vi "create.messages.for.testing.vi"(10 "Message.to.Create":refnum<class "MessageBase.lvclass">[](array[class]), 11 "Messages to Create":T1[](array[typedef])) -> (3 "Words.Out":u16[](array[numeric]) format="%.0x")   [LabVIEW 2020]
uses:
  Message.Spec.ctl
  pitch/oldMessageType.ctl
  pitch/AddOrder/AddOrderLong.Parameters.ctl
  pitch/Time/Time.Parameters.ctl
  pitch/SequencedUnitHeader/SequencedUnitHeader.Parameters.ctl
  pitch/ModifyOrder/ModifyOrderLong.Parameters.ctl
  pitch/MessageBase/MessageBase.lvclass
  pitch/SequencedUnitHeader/SequencedUnitHeader.lvclass
  pitch/Time/Time.lvclass
  pitch/AddOrder/AddOrderLong.lvclass
  pitch/ModifyOrder/ModifyOrderLong.lvclass
panel:
  out "size(s)":i32
  out "Remaining Bytes":u8[](array[numeric])
  out "Raw.Bytes.Out":u8[](array[numeric]) format="%.0x"
  out "Bytes.out (Visual)":u8[][](array[numeric]) format="%.0x"
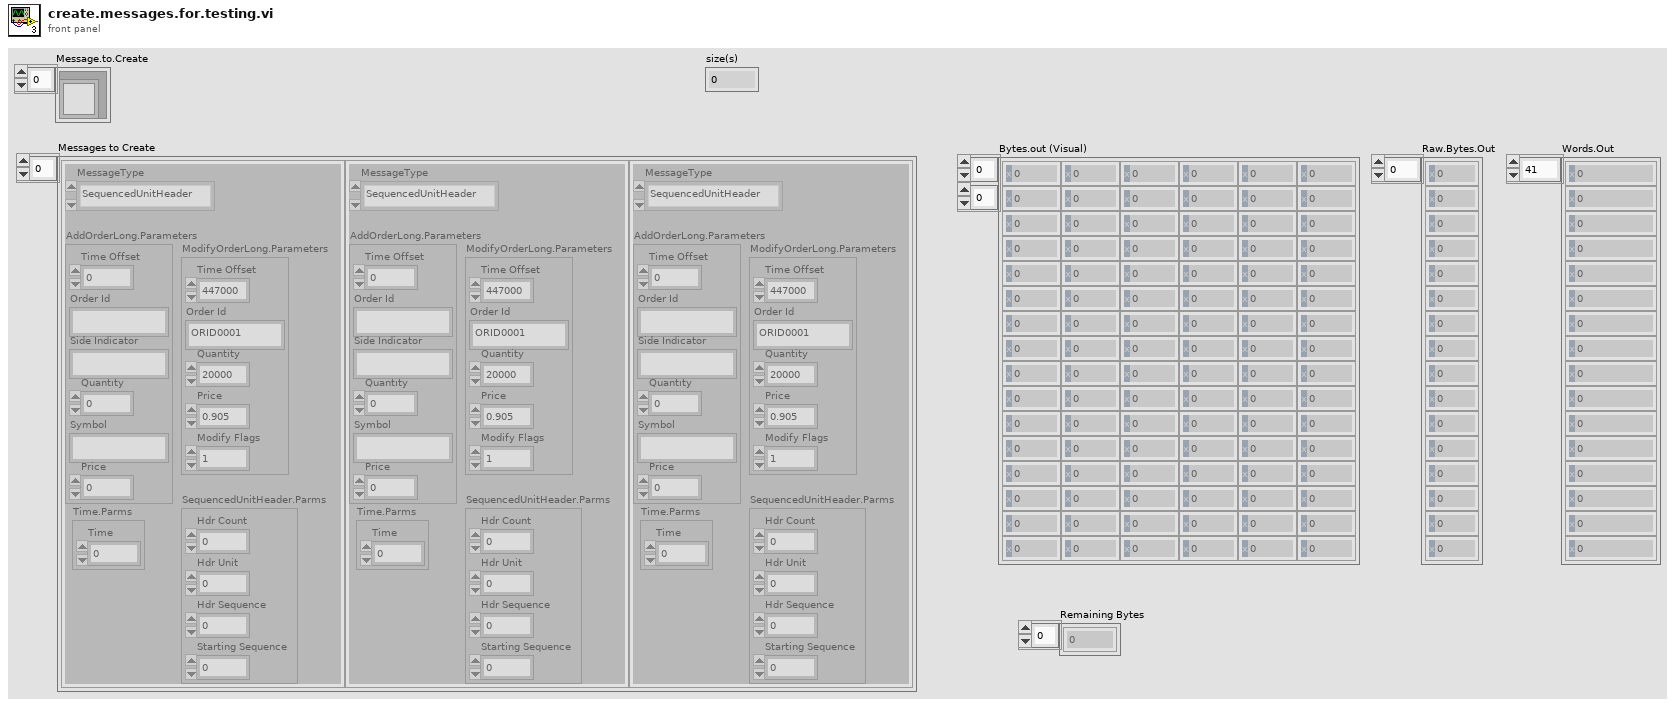
[diagram p1: front panel]
types:
  T1 = typedef "Message.Spec.ctl" = cluster{"MessageType":T2, "AddOrderLong.Parameters":T3, "Time.Parms":T4, "SequencedUnitHeader.Parms":T5, "ModifyOrderLong.Parameters":T6}
  T2 = typedef "oldMessageType.ctl" = enum16{"Time", "SequencedUnitHeader", "AddOrderLong", "AddOrderShort", "AddOrderExpanded", "ModifyOrderLong"}
  T3 = typedef "AddOrderLong.lvclass/AddOrderLong.Parameters.ctl" = cluster{"Time Offset":u32, "Order Id":string, "Quantity":u32, "Symbol":string, "Side Indicator":string, "Price":dbl}
  T4 = typedef "Time.lvclass/Time.Parameters.ctl" = cluster{"Time":u32}
  T5 = typedef "SequencedUnitHeader.lvclass/SequencedUnitHeader.Parameters.ctl" = cluster{"Hdr Count":u8, "Hdr Unit":u8, "Hdr Sequence":u32, "Starting Sequence":u32}
  T6 = typedef "ModifyOrderLong.lvclass/ModifyOrderLong.Parameters.ctl" = cluster{"Time Offset":u32, "Order Id":string, "Quantity":u32, "Price":dbl, "Modify Flags":u8}
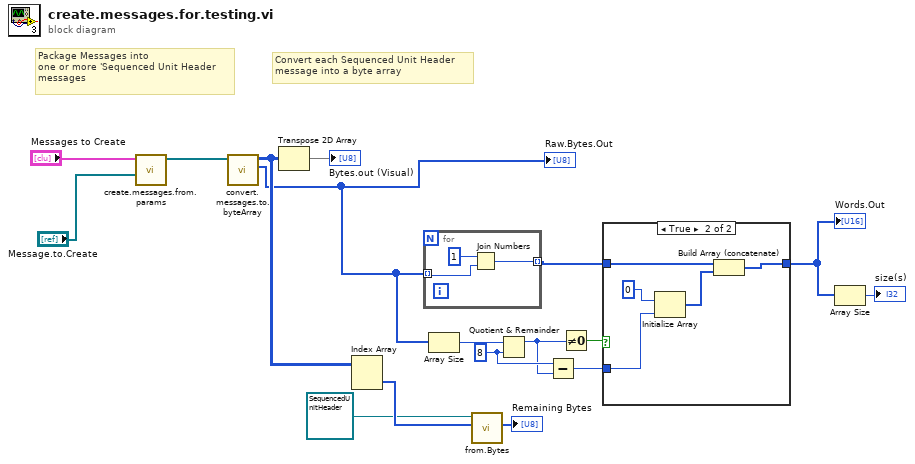
[diagram p0: block diagram]
diagram:
  w8 = 8 ("y")
  # "Convert each Sequenced Unit Header\nmessage into a byte array"
  # "Package Messages into\none or more 'Sequenced Unit Header\nmessages"
  n1 = call "create.messages.from.params.vi"("Message.to.Create"="Message.to.Create", "Messages to Create"="Messages to Create") -> ("Messages.Out"=w16:refnum<class "SequencedUnitHeader.lvclass">[])  [unwired: 9 in]
  n2 = call "convert.messages.to.byteArray.vi"("Messages.In"=w16) -> ("ByteArray.out"=w9:u8[], "2D.ByteArray.out"=w11:u8[][])  [unwired: 9 in]
  "Raw.Bytes.Out" <- w9
  n3 = Transpose 2D Array(2D array=w11) -> (transposed array=→"Bytes.out (Visual)":u8[][])
  n4 = Index Array(array=w11) -> (element=w14:u8[])  [unwired: 2 in]
  n5 = for {
    tunnel: w9 -> [w20] mode=indexing
    tunnel: [w18] -> w5 mode=indexing
    n6 = Join Numbers(hi=u8 1, lo=w20) -> ((hi.lo)=w18:u16)
  }
  n7 = Array Size(array=w9) -> (size(s)=w10:i32)
  n8 = call-dynamic "from.Bytes.vi"("Bytes.In"=w14, "SequencedUnitHeader in"=refnum<class "SequencedUnitHeader.lvclass"> refnum ("SequencedUnitHeader.lvclass")) -> ("Remaining Bytes"=→"Remaining Bytes":u8[])  [unwired: 7 in, 2 out]
  n9 = Quotient & Remainder(x=w10, y=w8) -> (x-y*floor(x/y)=w7:i32)  [unwired: 1 out]
  n10 = Subtract(x=w8, y=w7) -> (x-y=w4:i32)
  n11 = Not Equal To 0?(x=w7) -> (x != 0?=w6:bool)
  n12 = case shown="True" w6 {
    tunnel: w5 -> [w21 w25]
    tunnel: [w21 w24] -> w3
    tunnel: w4 -> [_ w22]
    frame False {
    }
    frame True {
      n13 = Initialize Array(u16 0, w22) -> (w26:u16[])
      n14 = Build Array (concatenate)(w25, w26) -> (w24:u16[])
    }
  }
  "Words.Out" <- w3
  n15 = Array Size(array=w3) -> (size(s)=→"size(s)":i32)
